vi "Create.vi"(8 "error in (no error)":errorcluster, 11 "Bar in":refnum<class "Bar.lvclass">) -> (0 "error out":errorcluster, 3 "Bar out":refnum<class "Bar.lvclass">)   [LabVIEW 2015, in "Simple Progress Bar.lvlib" / "Bar.lvclass"]
doc: "Create a new instance of progress bar. You have to call this VI for all independant instances you need."
uses:
  Bar.lvclass
  Bar.lvclass/Bar.ctl
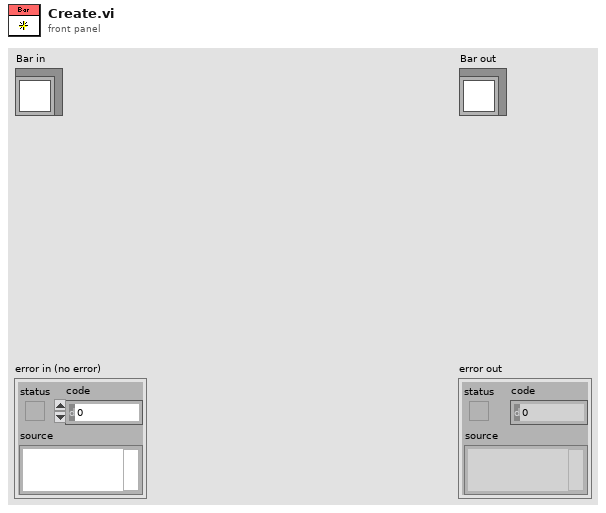
[diagram p1: front panel]
types:
  T1 = typedef "Simple Progress Bar.lvlib/Process Events.ctl" = cluster{"Explorer":refnum<user-event>, "Finished":refnum<user-event>, "Aborted":refnum<user-event>, "New Job":refnum<user-event>, "Item Status":refnum<user-event>, "Item Progression":refnum<user-event>, "Error":refnum<user-event>}
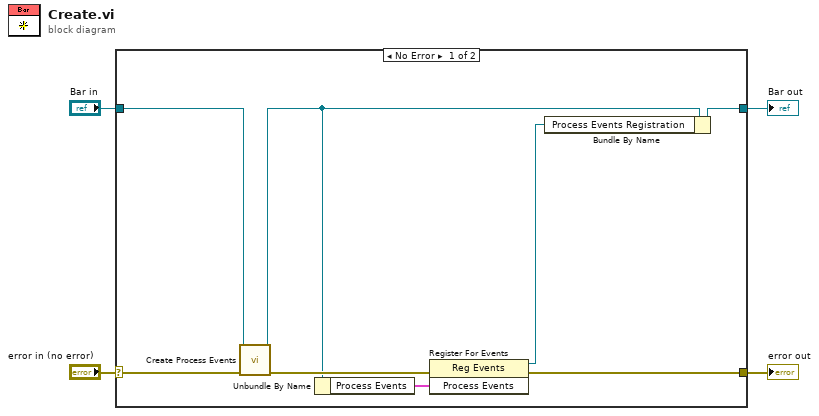
[diagram p0: block diagram]
diagram:
  n1 = case shown="No Error" "error in (no error)" {
    selector: "error in (no error)" -> [w12 w14]
    tunnel: [w9 w14] -> w3
    tunnel: [w7 w13] -> w1
    tunnel: "Bar in" -> [w11 w13]
    frame No Error {
      n2 = call "Create Process Events.vi"("error in (no error)"=w12, "Bar in"=w11) -> ("error out"=w10:errorcluster, "Bar out"=w8:refnum<class "Bar.lvclass">)  [unwired: 8 in]
      n3 = Unbundle By Name(w8) -> ("Process Events"=w6:T1)
      n4 = register-events(error in=w10, w6) -> (reference out=w5:refnum<event-registration>, error out=w9:errorcluster)  [unwired: 1 in]
      n5 = Bundle By Name(cluster=w8, "Process Events Registration"=w5) -> (w7:refnum<class "Bar.lvclass">)
    }
    frame Error {
    }
  }
  "error out" <- w3
  "Bar out" <- w1
